vi "Write uL_ms.vi"(8 "error in (no error)":errorcluster, 10 "uL/ms":dbl, 11 "TTLWaterDelivery in":refnum<class "TTLWaterDelivery.lvclass">) -> (0 "error out":errorcluster, 3 "TTLWaterDelivery out":refnum<class "TTLWaterDelivery.lvclass">)   [LabVIEW 2020, in "TTLWaterDelivery.lvclass"]
uses:
  TTLWaterDelivery.lvclass
  TTLWaterDelivery.lvclass/TTLWaterDelivery.ctl
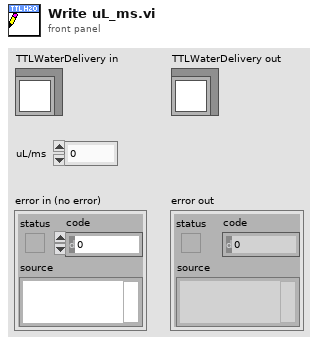
[diagram p1: front panel]
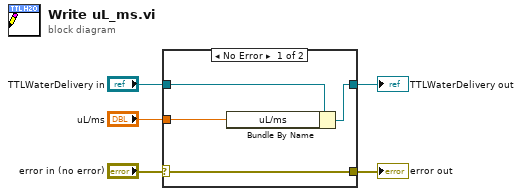
[diagram p0: block diagram]
diagram:
  n1 = case shown="No Error" "error in (no error)" {
    selector: "error in (no error)" -> [w9 w10]
    tunnel: [w9 w10] -> w4
    tunnel: [w7 w11] -> w2
    tunnel: "TTLWaterDelivery in" -> [w8 w11]
    tunnel: "uL/ms" -> [w6 _]
    frame No Error {
      n2 = Bundle By Name(cluster=w8, "uL/ms"=w6) -> (w7:refnum<class "TTLWaterDelivery.lvclass">)
    }
    frame Error {
    }
  }
  "error out" <- w4
  "TTLWaterDelivery out" <- w2
